vi "Reconnect.vi"(8 "error in (no error)":errorcluster, 11 "navX - Interface in":refnum<class "navX - Interface.lvclass">) -> (0 "error out":errorcluster, 3 "navX - Interface out":refnum<class "navX - Interface.lvclass">)   [LabVIEW 2015, in "navX Library v3.lvlib" / "navX - Interface.lvclass"]
uses:
  navX - Interface.lvclass
  navX - Interface.lvclass/navX - Interface.ctl
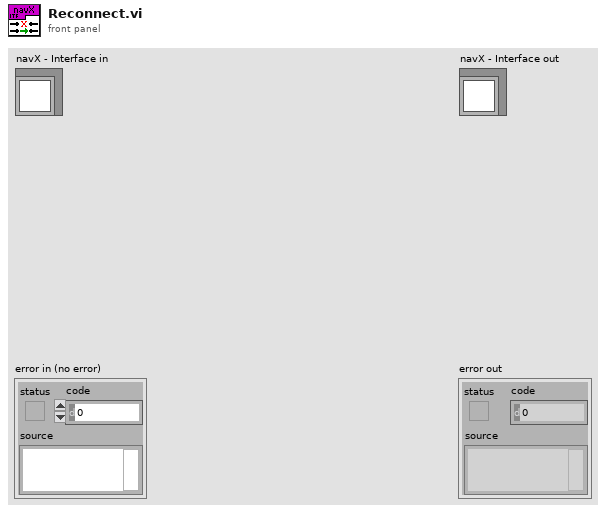
[diagram p1: front panel]
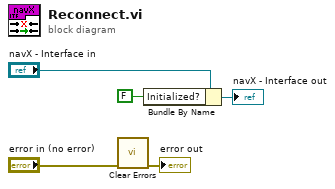
[diagram p0: block diagram]
diagram:
  n1 = call <vilib>:"Clear Errors.vi"("error in (no error)"="error in (no error)") -> ("error out"=→"error out":errorcluster)  [unwired: 5 in, 1 out]
  n2 = Bundle By Name(cluster="navX - Interface in", "Initialized?"=FALSE) -> (→"navX - Interface out":refnum<class "navX - Interface.lvclass">)
